vi "Presynthesize.vi"(0 "Moving Ripple Noise in":refnum<class "Moving Ripple Noise.lvclass">, 5 "Channel in":refnum<class "Channel.lvclass">, 11 "error in (no error)":errorcluster) -> (4 "Moving Ripple Noise out":refnum<class "Moving Ripple Noise.lvclass">, 6 "Channel out":refnum<class "Channel.lvclass">, 15 "error out":errorcluster)   [LabVIEW 2020, in "Moving Ripple Noise.lvclass"]
uses:
  Moving Ripple Noise.lvclass
  Channel/Channel.lvclass
  Waveform/Waveform.lvclass
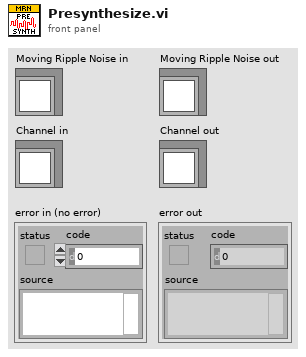
[diagram p1: front panel]
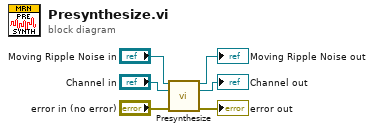
[diagram p0: block diagram]
diagram:
  n1 = call-parent "Presynthesize.vi"("Waveform in"="Moving Ripple Noise in", "Channel in"="Channel in", "error in (no error)"="error in (no error)") -> ("Waveform out"=→"Moving Ripple Noise out":refnum<class "Moving Ripple Noise.lvclass">, "Channel out"=→"Channel out":refnum<class "Channel.lvclass">, "error out"=→"error out":errorcluster)  [unwired: 10 in]
